vi "Convert Coords to Greyscale Selector.vi"(8 "error in (no error)":errorcluster, 10 "Coords in (Panel)":T1, 11 "ColorSelector in":refnum<class "ColorSelector.lvclass">) -> (0 "error out":errorcluster, 2 "Coords in (Control)":T1, 3 "ColorSelector (dup)":refnum<class "ColorSelector.lvclass">)   [LabVIEW 2015]
uses:
  <vilib>/Utility/miscctls.llb/LVPoint32TypeDef.ctl
  ColorSelector.lvclass
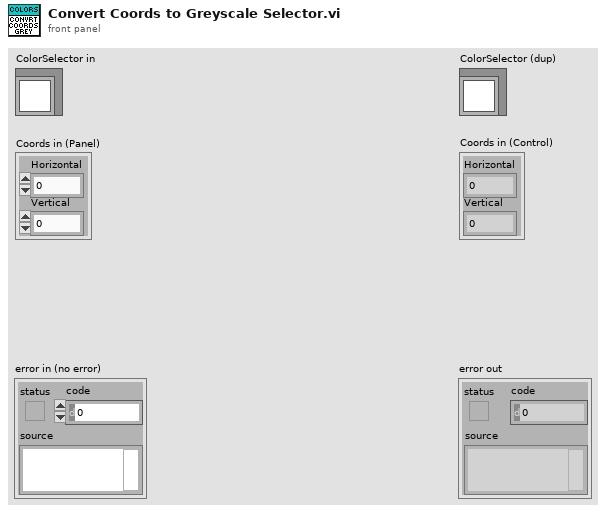
[diagram p1: front panel]
types:
  T1 = typedef "LVPoint32TypeDef.ctl" = cluster{"Horizontal":i32, "Vertical":i32}
  T2 = typedef "LVBoundsTypeDef.ctl" = cluster{"Width":u32, "Height":u32}
  T3 = typedef "LVPointTypeDef.ctl" = cluster{"Horizontal":i16, "Vertical":i16}
  T4 = typedef "LVPositionTypeDef.ctl" = cluster{"Left":i32, "Top":i32}
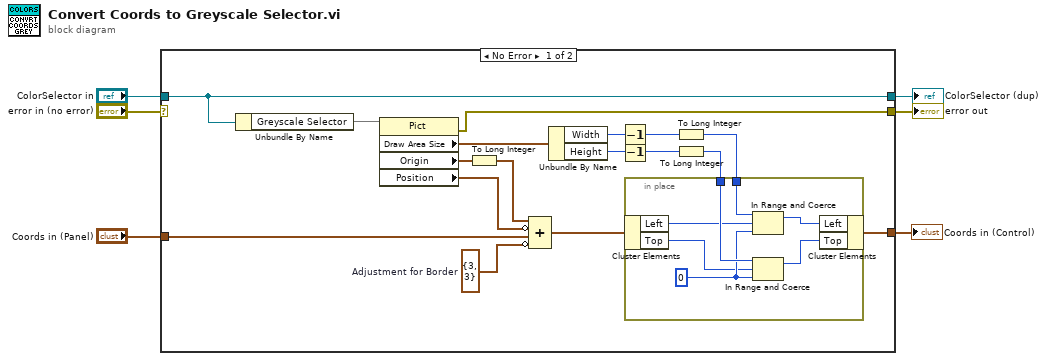
[diagram p0: block diagram]
diagram:
  n1 = case shown="No Error" "error in (no error)" {
    selector: "error in (no error)" -> [_ w33]
    tunnel: [w11 w33] -> w5
    tunnel: [w23 w32] -> w3
    tunnel: "ColorSelector in" -> [w23 w32]
    tunnel: "Coords in (Panel)" -> [w10 w31]
    tunnel: [w9 w31] -> w1
    frame No Error {
      w15 = T1 {"Horizontal"=3, "Vertical"=3}  # Adjustment for Border
      n2 = Unbundle By Name(w23) -> ("Greyscale Selector"=w12)
      n3 = property on="Property Node" class="Pict"(reference=w12) -> (error out=w11:errorcluster, "Draw Area Size"=w16:T2, "Origin"=w13:T3, "Position"=w14:T4)  [unwired: 1 in, 1 out]
      n4 = To Long Integer(number=w13) -> (32bit integer=w21:cluster{"Horizontal":i32, "Vertical":i32})
      n5 = Compound Arithmetic op=ADD(w21, invert w14, w10, invert w15) -> (w22:T4)
      n6 = Unbundle By Name(w16) -> ("Width"=w17:u32, "Height"=w18:u32)
      n7 = Decrement(x=w17) -> (x-1=w8:u32)
      n8 = Decrement(x=w18) -> (x-1=w7:u32)
      n9 = To Long Integer(number=w8) -> (32bit integer=w19:i32)
      n10 = To Long Integer(number=w7) -> (32bit integer=w20:i32)
      n11 = in-place {
        in-place-border: w19 -> [w30]
        in-place-border: w20 -> [w29]
        w28 = 0 ("lower limit")
        n12 = in-place-cluster #1(w22) -> ("Left"=w27:i32, "Top"=w26:i32)
        n13 = In Range and Coerce(upper limit=w30, x=w27, lower limit=w28) -> (coerced(x)=w25:i32)  [unwired: 1 out]
        n14 = In Range and Coerce(upper limit=w29, x=w26, lower limit=w28) -> (coerced(x)=w24:i32)  [unwired: 1 out]
        n15 = in-place-cluster #1("Left"=w25, "Top"=w24) -> (w9:T4)
      }
    }
    frame Error {
    }
  }
  "error out" <- w5
  "ColorSelector (dup)" <- w3
  "Coords in (Control)" <- w1
